vi "Initialize.vi"(8 "error in (no error)":errorcluster, 11 "TestStand Result Handler in":refnum<class "TestStand Result Handler.lvclass">) -> (0 "error out":errorcluster, 3 "TestStand Result Handler out":refnum<class "TestStand Result Handler.lvclass">)   [LabVIEW 2020, in "Astemes_CSVReportPlugin.lvlib" / "TestStand Result Handler.lvclass"]
uses:
  TestStand Result Handler.lvclass
  TestStand Result Handler.lvclass/TestStand Result Handler.ctl
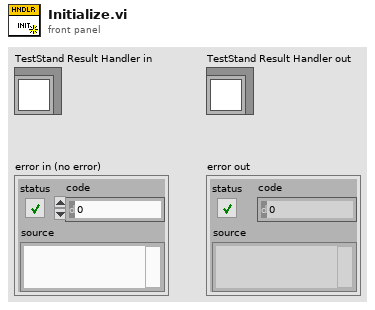
[diagram p1: front panel]
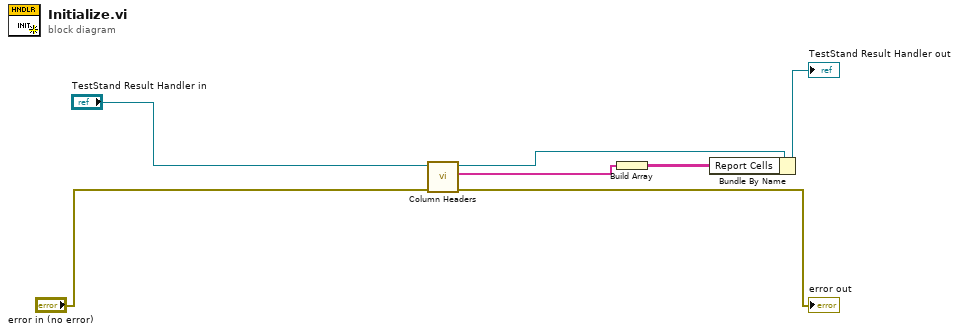
[diagram p0: block diagram]
diagram:
  n1 = call-dynamic "Column Headers.vi"("error in (no error)"="error in (no error)", "TestStand Result Handler in"="TestStand Result Handler in") -> ("error out"=→"error out":errorcluster, "Array"=w2:string[], "TestStand Result Handler out"=w5:refnum<class "TestStand Result Handler.lvclass">)  [unwired: 7 in]
  n2 = Build Array(w2) -> (w3:string[][])
  n3 = Bundle By Name(cluster=w5, "Report Cells"=w3) -> (→"TestStand Result Handler out":refnum<class "TestStand Result Handler.lvclass">)
